vi "Write State.vi"(8 "error in (no error)":errorcluster, 10 "Set":T1, 11 "Shutter in":refnum<class "Shutter.lvclass">) -> (0 "error out":errorcluster, 3 "Shutter out":refnum<class "Shutter.lvclass">)   [LabVIEW 2016, in "Shutter.lvclass"]
uses:
  Shutter.lvclass
  Controls/Shutter States.ctl
  Shutter.lvclass/Shutter.ctl
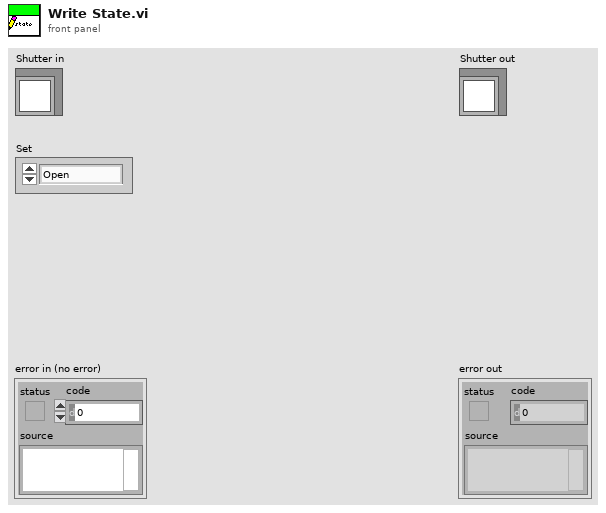
[diagram p1: front panel]
types:
  T1 = typedef "Shutter States.ctl" = enum16{"Open", "Close", "Wait", "Off", "Arm", "Idle"}
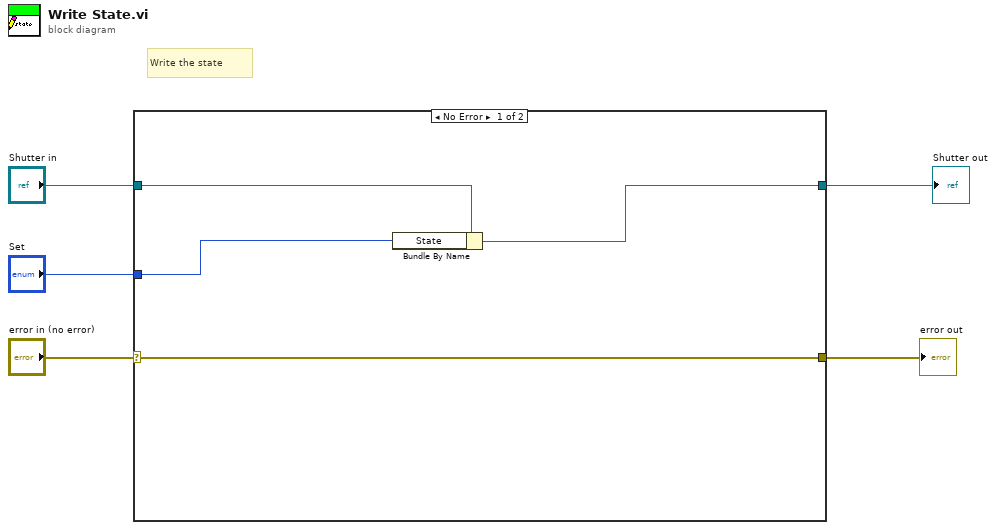
[diagram p0: block diagram]
diagram:
  # "Write the state"
  n1 = case shown="No Error" "error in (no error)" {
    selector: "error in (no error)" -> [w9 w10]
    tunnel: [w9 w10] -> w4
    tunnel: [w6 w11] -> w2
    tunnel: "Shutter in" -> [w7 w11]
    tunnel: "Set" -> [w8 _]
    frame No Error {
      n2 = Bundle By Name(cluster=w7, "State"=w8) -> (w6:refnum<class "Shutter.lvclass">)
    }
    frame Error {
    }
  }
  "error out" <- w4
  "Shutter out" <- w2
